vi "RT Driver VI.vi"(7 "Operation":T1, 11 "Device Reference in":T2 format="%.0x") -> (0 "Error Code":i32)   [LabVIEW 2015, in "Inline Async Example Engine.lvlib"]
uses:
  Inline Async Example Engine.lvlib
  <vilib>/NI Veristand/Custom Device API/Custom Device Item Ref.ctl
  <vilib>/NI Veristand/Custom Device API/Hardware Interface Driver VI Operation.ctl
  Inline Async APIs/VS Inline Async API/VS Inline Async API.lvclass
  Inline Async APIs/VS Inline Async API/VS Inline Async API.lvclass/VS Inline Async API.ctl
  Inline Async APIs/Data Access Engine/Data Access Engine.lvclass/Data Access Engine.ctl
  Inline Async APIs/Data Access Engine/Data/Write/Write.lvclass/Write.ctl
  Inline Async APIs/Data Access Engine/Data/ReadWrite/ReadWrite.lvclass/ReadWrite.ctl
  Inline Async APIs/Data Access Engine/Data/Read/Read.lvclass/Read.ctl
  Inline Async APIs/VS Inline Async API/SubVIs/Create Trigger.vi
  Inline Async APIs/VS Inline Async API/SubVIs/Connect to Error Handles.vi
  Inline Async APIs/Data Access Engine/Data/ReadWrite/ReadWrite.EngineData.vi
  Inline Async APIs/Data Access Engine/Data/Write/Write.EngineData.vi
  Inline Async APIs/Data Access Engine/Data/Read/Read.EngineData.vi
  <vilib>/NI Veristand/Custom Device API/NI VeriStand - Get Channel Value by Data Reference.vi
  <vilib>/NI Veristand/Custom Device API/NI VeriStand - Set Channel Value by Data Reference.vi
  <vilib>/NI Veristand/Custom Device API/NI VeriStand - Get Channel Values by Block Data Reference.vi
  Example.Async.vi
  <vilib>/NI Veristand/Custom Device API/Get Item Property (Variant).vi
  Inline Async APIs/VS Inline Async API/Display and Log Process.vi
  Inline Async APIs/VS Inline Async API/SubVIs/Initialize Global Stop.vi
  Inline Async APIs/VS Inline Async API/SubVIs/Run Process.vi
  <vilib>/Utility/error.llb/Error Cluster From Error Code.vi
  <vilib>/NI Veristand/Custom Device API/Global Data Refs.vi
  <vilib>/NI Veristand/Custom Device API/Custom Device API.lvlib
  Inline Async APIs/Data Access Engine/Data Access Engine.lvclass
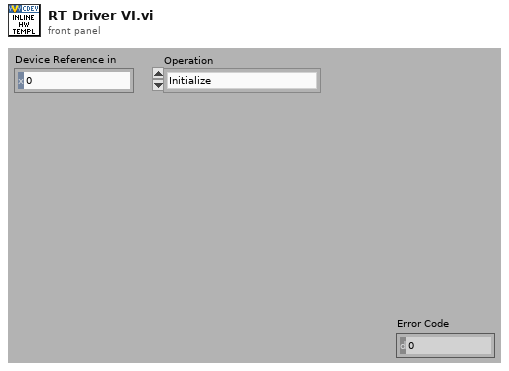
[diagram p1: front panel]
types:
  T1 = typedef "Custom Device API.lvlib/Hardware Interface Driver VI Operation.ctl" = enum16{"Initialize", "Start", "Read Data from HW", "Write Data to HW", "Close"}
  T2 = typedef "Custom Device API.lvlib/Custom Device Item Ref.ctl" = u64
  T3 = cluster{"Data Access Engine":refnum<class "Data Access Engine.lvclass">, "Async out":refnum<class "VS Inline Async API.lvclass">}
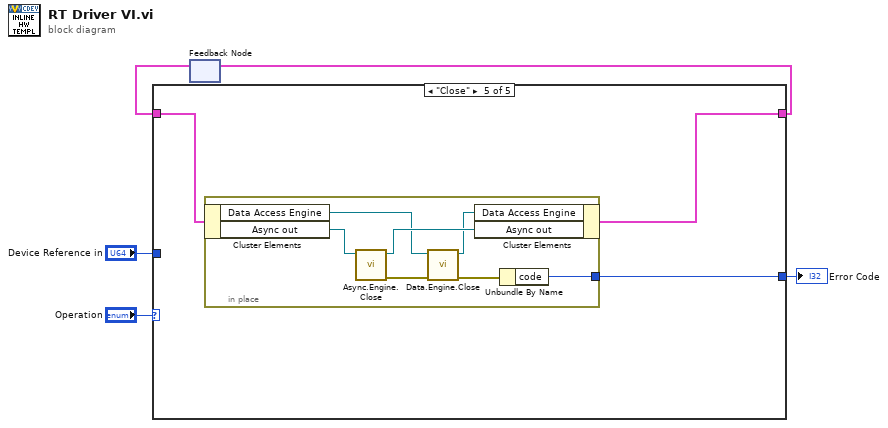
[diagram p0: block diagram]
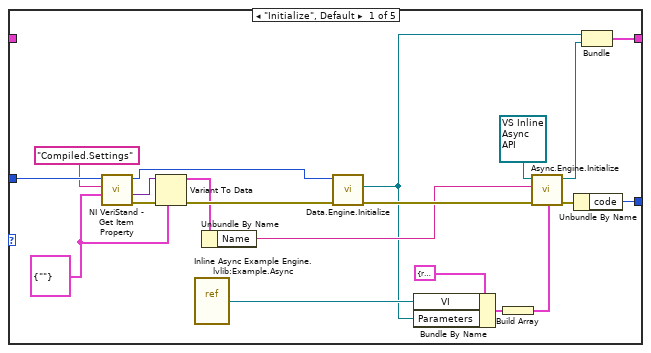
[diagram p2: hidden frame]
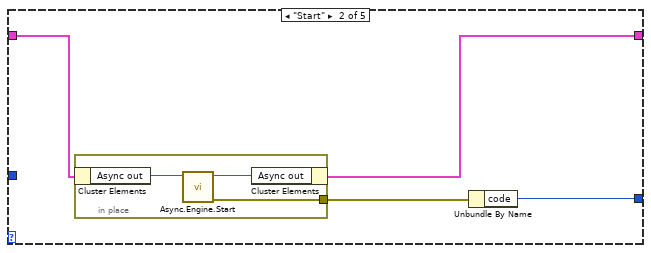
[diagram p3: hidden frame]
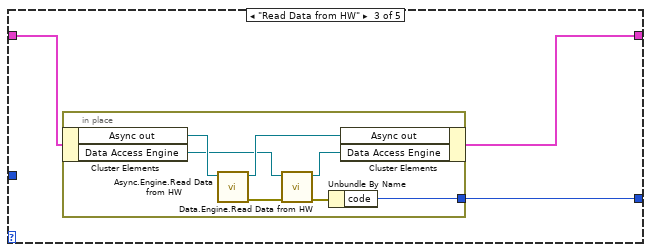
[diagram p4: hidden frame]
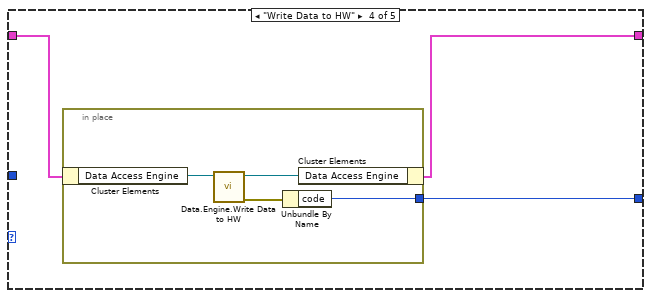
[diagram p5: hidden frame]
diagram:
  n1 = feedback #1() -> (w3:T3)  [unwired: 1 out]
  n2 = case shown="\"Close\"" "Operation" {
    tunnel: [w22 w26 w34 w43 w51] -> w4
    tunnel: w3 -> [_ w27 w35 w44 w52]
    tunnel: "Device Reference in" -> [w18 _ _ _ _]
    tunnel: [w25 w29 w33 w45 w50] -> w1
    frame "Initialize", Default {
      w9 = cluster{"Name":string} {"Name"=""}
      n3 = call-poly <vilib>:"NI VeriStand - Get Item Property.vi"("Default Value"=w9, "Property Name"="Compiled.Settings", "Item Ref in"=w18) -> ("error out"=w17:errorcluster, "Value"=w16:variant, "Item Ref out"=w7:T2)  [unwired: 5 in, 1 out]
      n4 = Variant To Data(error in=w17, type=w9, Variant=w16) -> (data=w11:cluster{"Name":string}, error out=w13:errorcluster)
      n5 = vi-ref "Inline Async Example Engine.lvlib:Example.Async.vi"() -> (w20:refnum<vi>)
      n6 = Unbundle By Name(w11) -> ("Name"=w10:string)
      n7 = call "Data.Engine.Initialize.vi"("error in"=w13, "Custom Device Ref"=w7) -> ("error out"=w12:errorcluster, "Data Access Engine"=w6:refnum<class "Data Access Engine.lvclass">)  [unwired: 7 in, 1 out]
      n8 = Bundle By Name(cluster=cluster{"VI":refnum<vi>, "Parameters":variant} {"VI"=refnum, "Parameters"=variant} ("Process"), "VI"=w20, "Parameters"=w6) -> (w19:cluster{"VI":refnum<vi>, "Parameters":variant})
      n9 = Build Array(w19) -> (w14:cluster{"VI":refnum<vi>, "Parameters":variant}[])
      n10 = call "Async.Engine.Initialize.vi"("error in (no error)"=w12, "Processes"=w14, "Name"=w10, "Async in"=refnum<class "VS Inline Async API.lvclass"> refnum) -> ("error out"=w8:errorcluster, "Async out"=w23:refnum<class "VS Inline Async API.lvclass">)  [unwired: 6 in]
      n11 = Unbundle By Name(w8) -> ("code"=w25:i32)
      n12 = Bundle("Data Access Engine"=w6, "Async out"=w23) -> (w22:T3)  [unwired: 1 in]
    }
    frame "Start" {
      n13 = in-place {
        in-place-border: [w30] -> w28
        n14 = in-place-cluster #2(w27) -> ("Async out"=w32:refnum<class "VS Inline Async API.lvclass">)
        n15 = call "Async.Engine.Start.vi"("VS Inline Async API in"=w32) -> ("error out"=w30:errorcluster, "VS Inline Async API out"=w31:refnum<class "VS Inline Async API.lvclass">)  [unwired: 9 in]
        n16 = in-place-cluster #2("Async out"=w31) -> (w26:T3)
      }
      n17 = Unbundle By Name(w28) -> ("code"=w29:i32)
    }
    frame "Read Data from HW" {
      n18 = in-place {
        in-place-border: [w38] -> w33
        n19 = in-place-cluster #3(w35) -> ("Async out"=w42:refnum<class "VS Inline Async API.lvclass">, "Data Access Engine"=w37:refnum<class "Data Access Engine.lvclass">)
        n20 = call "Async.Engine.Read Data from HW.vi"("Async in"=w42) -> ("error out"=w40:errorcluster, "Async out"=w41:refnum<class "VS Inline Async API.lvclass">)  [unwired: 9 in]
        n21 = call "Data.Engine.Read Data from HW.vi"("error in (no error)"=w40, "Data Access API in"=w37) -> ("error out"=w39:errorcluster, "Data Access API out"=w36:refnum<class "Data Access Engine.lvclass">)  [unwired: 8 in]
        n22 = Unbundle By Name(w39) -> ("code"=w38:i32)
        n23 = in-place-cluster #3("Async out"=w41, "Data Access Engine"=w36) -> (w34:T3)
      }
    }
    frame "Write Data to HW" {
      n24 = in-place {
        in-place-border: [w49] -> w45
        n25 = in-place-cluster #4(w44) -> ("Data Access Engine"=w47:refnum<class "Data Access Engine.lvclass">)
        n26 = call "Data.Engine.Write Data to HW.vi"("Data Access API in"=w47) -> ("error out"=w48:errorcluster, "Data Access API out"=w46:refnum<class "Data Access Engine.lvclass">)  [unwired: 9 in]
        n27 = Unbundle By Name(w48) -> ("code"=w49:i32)
        n28 = in-place-cluster #4("Data Access Engine"=w46) -> (w43:T3)
      }
    }
    frame "Close" {
      n29 = in-place {
        in-place-border: [w57] -> w50
        n30 = in-place-cluster #5(w52) -> ("Data Access Engine"=w54:refnum<class "Data Access Engine.lvclass">, "Async out"=w59:refnum<class "VS Inline Async API.lvclass">)
        n31 = call "Async.Engine.Close.vi"("Async in"=w59) -> ("error out"=w56:errorcluster, "Async out"=w58:refnum<class "VS Inline Async API.lvclass">)  [unwired: 9 in]
        n32 = call "Data.Engine.Close.vi"("error in (no error)"=w56, "Data Access API in"=w54) -> ("error out"=w55:errorcluster, "Data Access API out"=w53:refnum<class "Data Access Engine.lvclass">)  [unwired: 8 in]
        n33 = in-place-cluster #5("Data Access Engine"=w53, "Async out"=w58) -> (w51:T3)
        n34 = Unbundle By Name(w55) -> ("code"=w57:i32)
      }
    }
  }
  "Error Code" <- w1
  n35 = feedback-in #1(w4) -> ()
